vi "Error handling.vi"(8 "error in (no error)":errorcluster) -> (0 "error out":errorcluster)   [LabVIEW 2023]
doc: "Use this template to build a VI to use as a subVI."
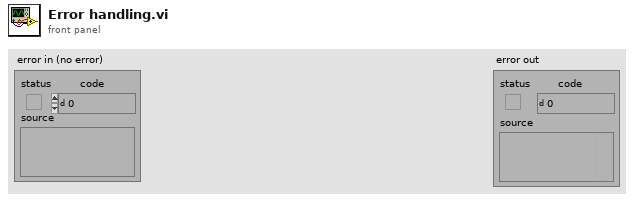
[diagram p1: front panel]
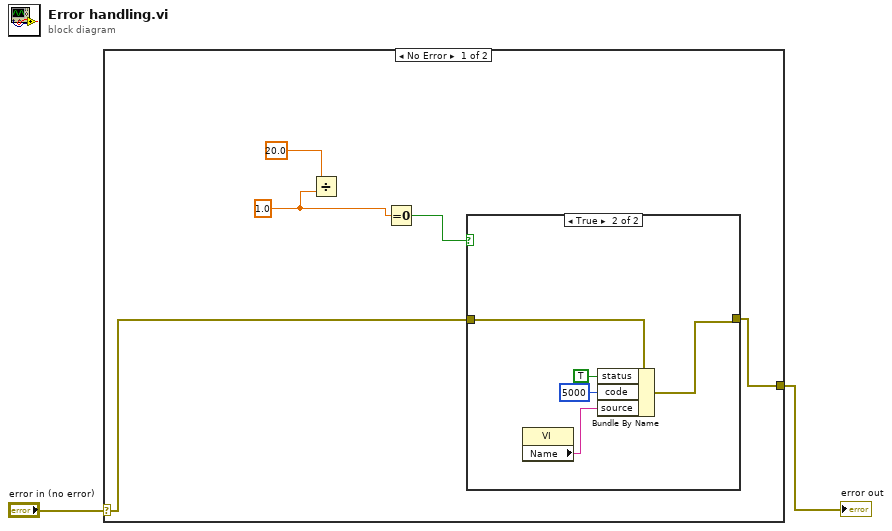
[diagram p0: block diagram]
diagram:
  n1 = case shown="No Error" "error in (no error)" {
    selector: "error in (no error)" -> [w4 w14]
    tunnel: [w3 w14] -> w1
    frame No Error {
      w6 = 1.0 ("y")
      n2 = Divide(x=20.0 ("x/y"), y=w6) -> ()  [unwired: 1 out]
      n3 = Equal To 0?(x=w6) -> (x = 0?=w5:bool)
      n4 = case shown="True" w5 {
        tunnel: w4 -> [w8 w13]
        tunnel: [w8 w12] -> w3
        frame False {
          # "kein Fehler"
        }
        frame True {
          n5 = property class="VI"() -> ("Name"=w9:string)  [unwired: 2 in, 2 out]
          n6 = Bundle By Name "Bundle By Name"(cluster=w13, "status"=TRUE, "code"=5000, "source"=w9) -> (w12:errorcluster)
        }
      }
    }
    frame Error {
    }
  }
  "error out" <- w1
